vi "unstable-detector.vi"(8 "x-max":sgl, 11 "x(k)":sgl) -> (2 "x >= y?":bool)   [LabVIEW 2015]
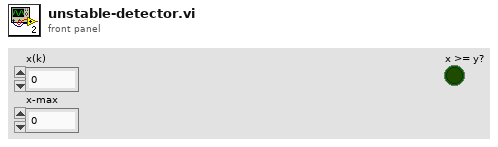
[diagram p1: front panel]
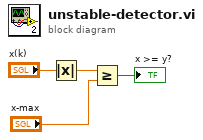
[diagram p0: block diagram]
diagram:
  n1 = Absolute Value(x="x(k)") -> (abs(x)=w4:sgl)
  n2 = Greater Or Equal?(x=w4, y="x-max") -> (x >= y?=→"x >= y?":bool)
